vi "mjquadraticcase.vi"() -> ()   [LabVIEW 2024]
panel:
  out "conditions\ncond":string
  out "root2":dbl
  out "root1":dbl
  in  "c":dbl
  in  "b":dbl
  in  "a":dbl
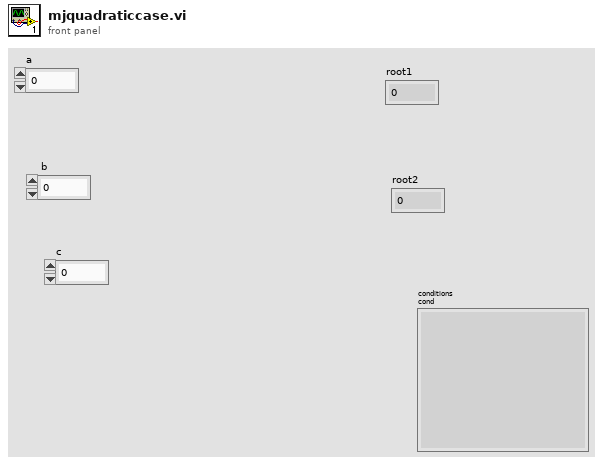
[diagram p1: front panel]
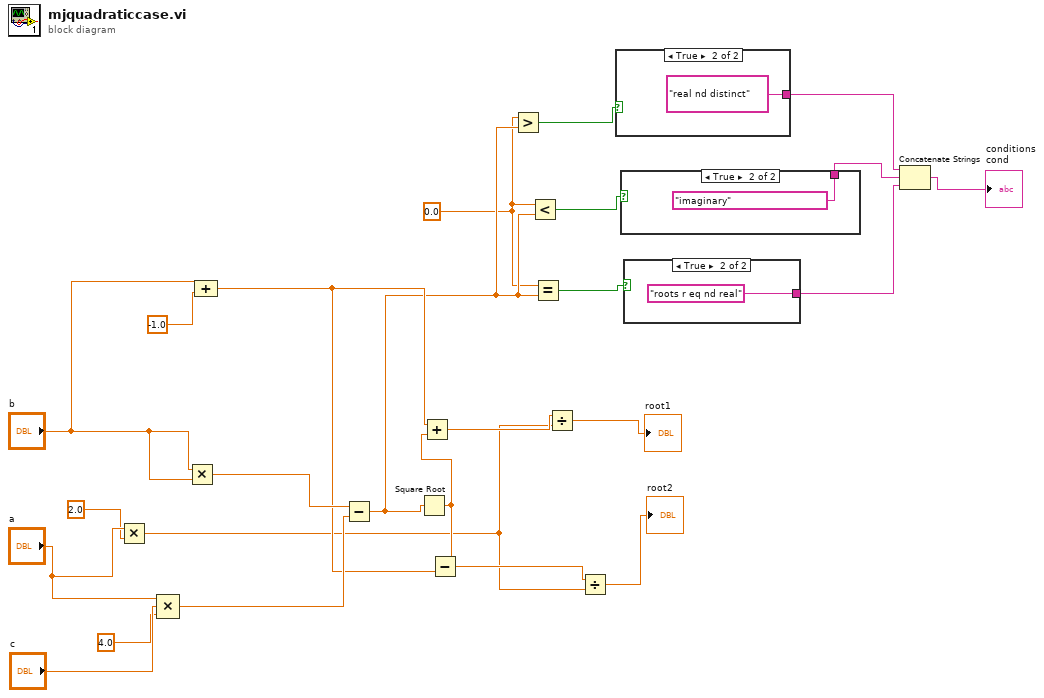
[diagram p0: block diagram]
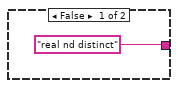
[diagram p4: hidden frame]
diagram:
  w9 = 0.0
  n1 = Multiply(x="a", y=2.0) -> (x*y=w13:dbl)
  n2 = Compound Arithmetic op=MULTIPLY("a", "c", 4.0) -> (w22:dbl)
  n3 = Multiply(x="b", y="b") -> (x*y=w24:dbl)
  n4 = Compound Arithmetic op=ADD("b", -1.0) -> (w18:dbl)
  n5 = Subtract(x=w24, y=w22) -> (x-y=w10:dbl)
  n6 = Square Root(x=w10) -> (sqrt(x)=w19:dbl)
  n7 = Add(x=w18, y=w19) -> (x+y=w17:dbl)
  n8 = Subtract(x=w19, y=w18) -> (x-y=w16:dbl)
  n9 = Greater?(x=w9, y=w10) -> (0:w8:bool)
  n10 = Less?(x=w9, y=w10) -> (x < y?=w7:bool)
  n11 = Equal?(x=w9, y=w10) -> (x = y?=w6:bool)
  n12 = Divide(x=w17, y=w13) -> (x/y=→"root1":dbl)
  n13 = Divide(x=w16, y=w13) -> (x/y=→"root2":dbl)
  n14 = case shown="True" w8 {
    tunnel: ["real nd distinct" "real nd distinct"] -> w5
    frame False {
    }
    frame True {
    }
  }
  n15 = case shown="True" w7 {
    tunnel: [_ "imaginary"] -> w2
    frame False {
    }
    frame True {
    }
  }
  n16 = case shown="True" w6 {
    tunnel: [_ "roots r eq nd real"] -> w1
    frame False {
    }
    frame True {
    }
  }
  n17 = Concatenate Strings(w5, w2, w1) -> (→"conditions\ncond":string)
